vi "Robot_line_path.vi"() -> ()   [LabVIEW 2011]
uses:
  <vilib>/NXT/Block Support/NXT_InputPort.ctl
  <vilib>/NXT/Subs/LVHSConnector.ctl
  <vilib>/NXT/Subs/MotorOutput.ctl
  <vilib>/NXT/Dual Mode Library/Motors/Rotation.vi
  <vilib>/NXT/Dual Mode Library/Sensors/Light_On.vi
  <vilib>/NXT/Dual Mode Library/Motors/MotorOn.vi
panel:
  in  "Threshold":i16
  out "Scaled Value":i16
  out "Distance (cm)":i16
  in  "y":dbl(knob) scale=75.0..-75.0
  in  "x":dbl
  out "Right Motor Rotation":i32 caption="Angle of Rotation"
  out "Left Motor Rotation":i32 caption="Angle of Rotation"
  in  "Ultrasonic Port":T1=3 caption="Port (Port 4)" items=["Port 1", "Port 2", "Port 3", "Port 4"]
  in  "Light Port":T1=2 caption="Port (Port 3)" items=["Port 1", "Port 2", "Port 3", "Port 4"]
  in  "stop":bool
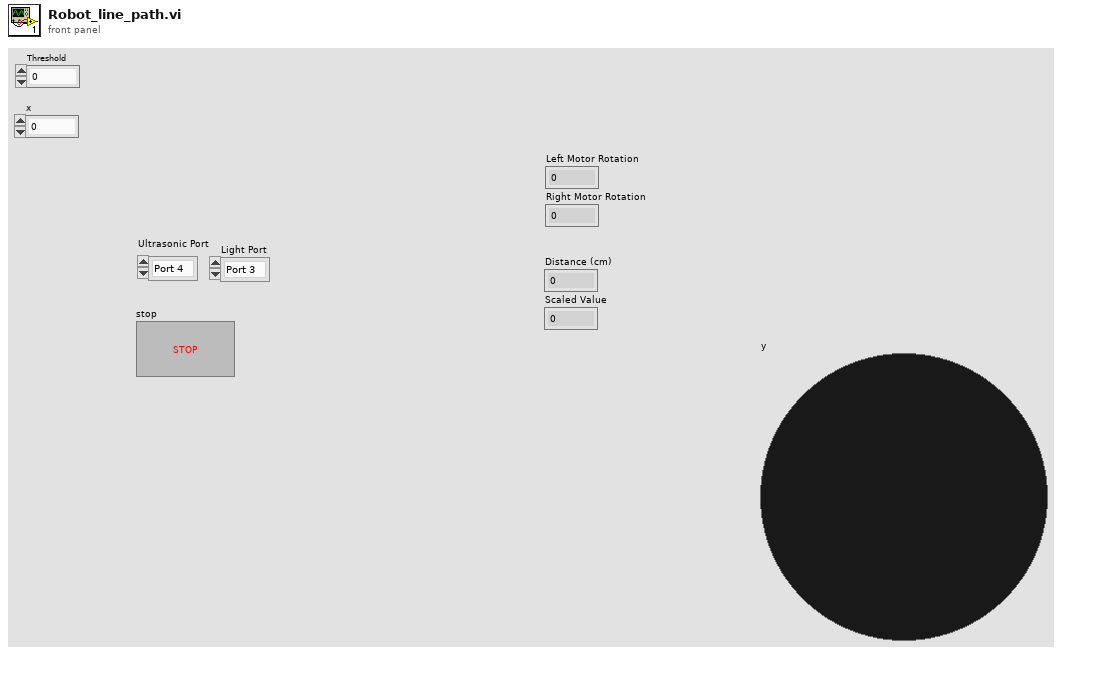
[diagram p1: front panel]
types:
  T1 = typedef "NXT_InputPort.ctl" = u8
  T2 = typedef "LVHSConnector.ctl" = cluster{"Hardware":string, "Flattened String":string}
  T3 = typedef "MotorOutput.ctl" = u8
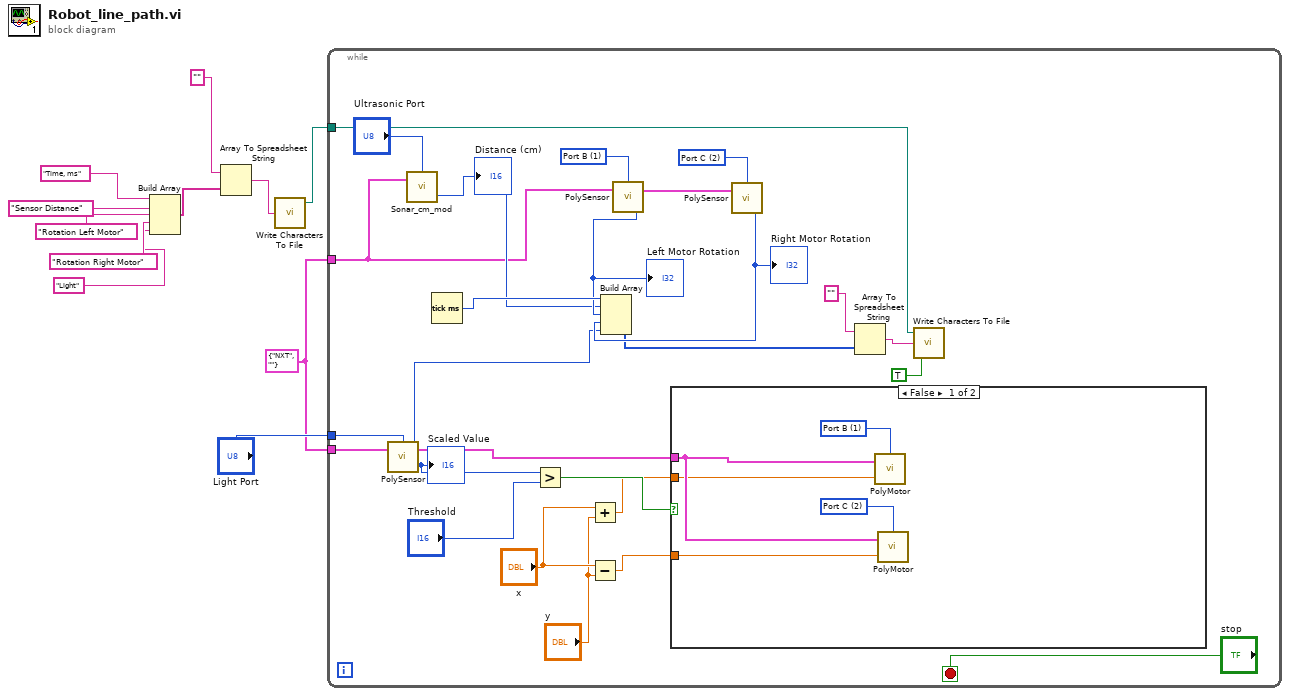
[diagram p0: block diagram]
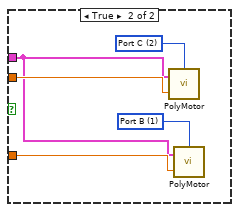
[diagram p2: hidden frame]
diagram:
  w1 = T2 {"Hardware"="NXT", "Flattened String"=""} ("NXT")
  n1 = Build Array("Time, ms" ("element"), "Sensor Distance" ("element"), "Rotation Left Motor", "Rotation Right Motor", "Light") -> (w7:string[])
  n2 = Array To Spreadsheet String(array=w7, 3:"" ("format string")) -> (spreadsheet string=w8:string)  [unwired: 1 in]
  n3 = call <vilib>:"Write Characters To File.vi"("character string"=w8) -> ("new file path (Not A Path if cancelled)"=w3:path)  [unwired: 4 in]
  n4 = while {
    tunnel: w3 -> [w27]
    tunnel: "Light Port" -> [w18]
    tunnel: w1 -> [w17]
    tunnel: w1 -> [w13]
    stop <- "stop" stop-if-true
    w14 = u8 2 items=["Port A", "Port B", "Port C"] ("Port (Port A)")
    w15 = u8 1 items=["Port A", "Port B", "Port C"] ("Port (Port A)")
    n5 = call-poly <vilib>:"PolySensor.vi"("NXT"=w17, "Port (Port 3)"=w18) -> ("Scaled Value"=w25:i16, "NXT"=w19:T2)  [unwired: 1 in]
    "Scaled Value" <- w25
    n6 = call <vilib>:"Sonar_cm_mod.vi"("NXT"=w13, "Port (Port 4)"="Ultrasonic Port") -> ("Distance (cm)"=w26:i16)  [unwired: 1 in, 1 out]
    "Distance (cm)" <- w26
    n7 = Tick Count (ms)() -> (millisecond timer value=w35:u32)
    n8 = Greater?(x=w25, y="Threshold") -> (0:w24:bool)
    n9 = Add(x="x", y="y") -> (x+y=w21:dbl)
    n10 = Subtract(x="x", y="y") -> (x-y=w20:dbl)
    n11 = call-poly <vilib>:"PolySensor.vi"("NXT"=w13, "Port (Port A)"=w15) -> ("Angle of Rotation"=w34:i32, "NXT"=w16:T2)  [unwired: 1 in]
    "Left Motor Rotation" <- w34
    n12 = case shown="False" w24 {
      tunnel: w19 -> [w39 w42]
      tunnel: w21 -> [w38 w44]
      tunnel: w20 -> [w37 w43]
      frame False {
        w40 = T3 2 items=["Port A"=0, "Port B"=1, "Port C"=2, "Ports A & B"=4, "Ports A & C"=5, "Ports B & C"=6, "All Ports"=3] ("Output Port (All Ports)")
        w41 = T3 1 items=["Port A"=0, "Port B"=1, "Port C"=2, "Ports A & B"=4, "Ports A & C"=5, "Ports B & C"=6, "All Ports"=3] ("Output Port (All Ports)")
        n13 = call-poly <vilib>:"PolyMotor.vi"("Power (75)"=w38, "NXT"=w39, "Output Port (All Ports)"=w41) -> ()  [unwired: 1 in, 1 out]
        n14 = call-poly <vilib>:"PolyMotor.vi"("Power (75)"=w37, "NXT"=w39, "Output Port (All Ports)"=w40) -> ()  [unwired: 1 in, 1 out]
      }
      frame True {
        w45 = T3 1 items=["Port A"=0, "Port B"=1, "Port C"=2, "Ports A & B"=4, "Ports A & C"=5, "Ports B & C"=6, "All Ports"=3] ("Output Port (All Ports)")
        w46 = T3 2 items=["Port A"=0, "Port B"=1, "Port C"=2, "Ports A & B"=4, "Ports A & C"=5, "Ports B & C"=6, "All Ports"=3] ("Output Port (All Ports)")
        n15 = call-poly <vilib>:"PolyMotor.vi"("Power (75)"=w44, "NXT"=w42, "Output Port (All Ports)"=w46) -> ()  [unwired: 1 in, 1 out]
        n16 = call-poly <vilib>:"PolyMotor.vi"("Power (75)"=w43, "NXT"=w42, "Output Port (All Ports)"=w45) -> ()  [unwired: 1 in, 1 out]
      }
    }
    n17 = call-poly <vilib>:"PolySensor.vi"("NXT"=w16, "Port (Port A)"=w14) -> ("Angle of Rotation"=w33:i32)  [unwired: 1 in, 1 out]
    "Right Motor Rotation" <- w33
    n18 = Build Array(w35, w26, w34, w33, w25) -> (w28:u32[])
    n19 = Array To Spreadsheet String(array=w28, 3:"" ("format string")) -> (spreadsheet string=w30:string)  [unwired: 1 in]
    n20 = call <vilib>:"Write Characters To File.vi"("append to file? (new file:F)"=TRUE ("convert eol? (no:F)"), "character string"=w30, "file path (dialog if empty)"=w27) -> ()  [unwired: 2 in, 1 out]
  }
